vi "Point&Path@Display2User__Parameter.vi"(1 "ParamterIn":string) -> (0 "ParamterOut":string)   [LabVIEW 2020]
panel:
  in  "Control":string(combo)
  in  "PointName":string(combo)
  in  "Confirm":bool
  # "Point&Path@Display2User $Point,$Control"
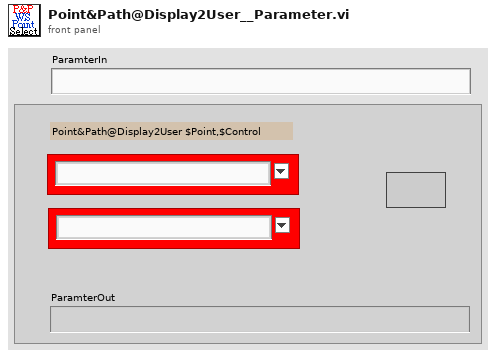
[diagram p1: front panel]
types:
  T1 = enum16{"Get", "UpdatePointS", "Init", "UpdateIndex", "GetCurrent&Index+1", "GetWithIndex", "ChkLast", "GetCurrent"}
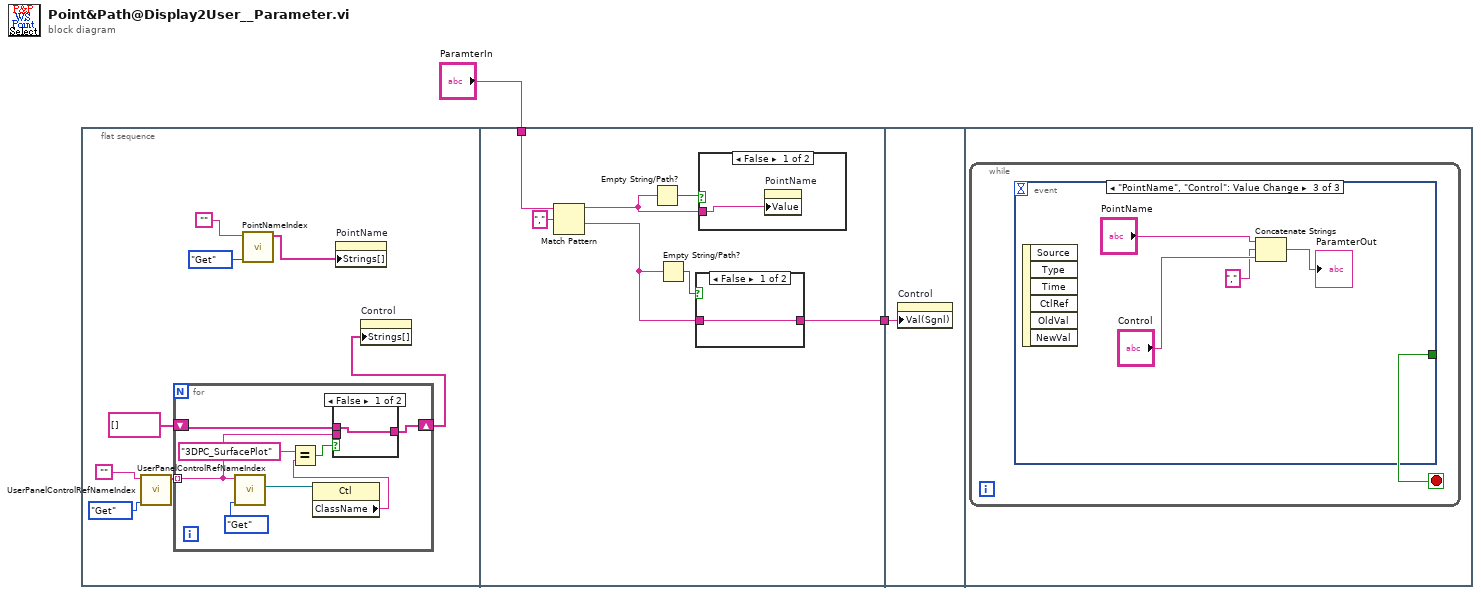
[diagram p0: block diagram]
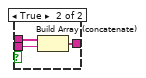
[diagram p2: hidden frame]
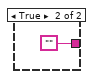
[diagram p3: hidden frame]
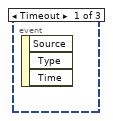
[diagram p5: hidden frame]
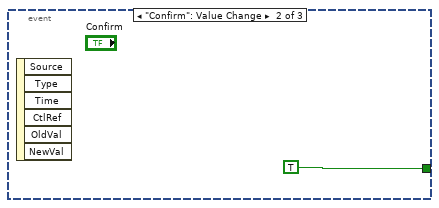
[diagram p6: hidden frame]
diagram:
  n1 = flat-sequence {
    tunnel: "ParamterIn" -> [w26]
    tunnel: [w27] -> w1
    tunnel: w1 -> [w33]
    frame #0 {
      n2 = call "UserPanelControlRefNameIndex.vi"("OP"=enum16{"Get", "Update", "Init"}."Get", "ControlName"="") -> ("ControlNameS"=w5:string[])  [unwired: 6 in, 3 out]
      n3 = for {
        tunnel: w5 -> [w12] mode=indexing
        shift-right: [w11] -> w3
        shift-left: string[] [] ("Strings []") -> [w13]
        n4 = call "UserPanelControlRefNameIndex.vi"("OP"=enum16{"Get", "Update", "Init"}."Get", "ControlName"=w12) -> ("ControlRefOut"=w17:refnum<vi>)  [unwired: 6 in, 3 out]
        n5 = property class="Ctl"(reference=w17) -> ("ClassName"=w15:string)  [unwired: 1 in, 2 out]
        n6 = Equal?(x="3DPC_SurfacePlot" ("Class Name"), y=w15) -> (x = y?=w14:bool)
        n7 = case shown="False" w14 {
          tunnel: w13 -> [w19 w22]
          tunnel: w12 -> [_ w21]
          tunnel: [w19 w20] -> w11
          frame False {
          }
          frame True {
            n8 = Build Array (concatenate)(w22, w21) -> (w20:string[])
          }
        }
      }
      n9 = call "PointNameIndex.vi"("OP"=T1."Get", "PointName"="") -> ("PointNameList"=w8:string[])  [unwired: 4 in, 5 out]
      n10 = property on="PointName" class="CmbBox"("Strings[]"=w8) -> ()  [unwired: 2 in, 2 out]
      n11 = property on="Control" class="CmbBox"("Strings[]"=w3) -> ()  [unwired: 2 in, 2 out]
    }
    frame #1 {
      n12 = Match Pattern(string=w26, regular expression="," ("search string")) -> (before substring=w23:string, after substring=w24:string)  [unwired: 1 in, 2 out]
      n13 = Empty String/Path?(string/path=w23) -> (empty?=w29:bool)
      n14 = Empty String/Path?(string/path=w24) -> (empty?=w28:bool)
      n15 = case shown="False" w28 {
        tunnel: [w30 ""] -> w27
        tunnel: w24 -> [w30 _]
        frame False {
        }
        frame True {
        }
      }
      n16 = case shown="False" w29 {
        tunnel: w23 -> [w32 _]
        frame False {
          n17 = property on="PointName" class="CmbBox"("Value"=w32) -> ()  [unwired: 2 in, 2 out]
        }
        frame True {
        }
      }
    }
    frame #2 {
      n18 = property on="Control" class="CmbBox"("Val(Sgnl)"=w33) -> ()  [unwired: 2 in, 2 out]
    }
    frame #3 {
      n19 = while {
        stop <- w34 stop-if-true
        n20 = event shown="[2] \"PointName\", \"Control\": Value Change" {
          selector: _ -> [_ _ _]
          dyn-events: _ -> [_ _ _]
          timeout: _ -> [_ _ _]
          tunnel: [_ TRUE _] -> w34
          event Timeout {
            n21 = event-data() -> ()  [unwired: 1 in, 3 out]
          }
          event "Confirm": Value Change {
            n22 = event-data() -> ()  [unwired: 1 in, 6 out]
          }
          event "PointName", "Control": Value Change {
            n23 = event-data() -> ()  [unwired: 1 in, 6 out]
            n24 = Concatenate Strings("PointName", ",", "Control") -> (→"ParamterOut":string)
          }
        }
      }
    }
  }
